vi "IRange Max Min.vi"(1 "resources":i32[](array[numeric])) -> (0 "disabled ranges":i32[](array[numeric]))   [LabVIEW 2022 SP3, in "EClib functions.lvlib"]
doc: "Builds an arrays of indices of the unavailable current ranges."
uses:
  EClib functions.lvlib
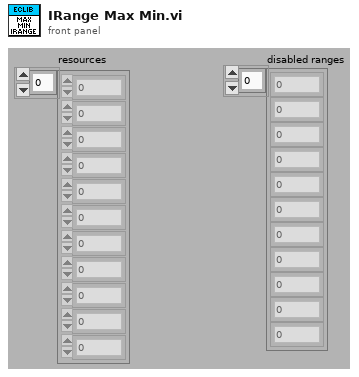
[diagram p1: front panel]
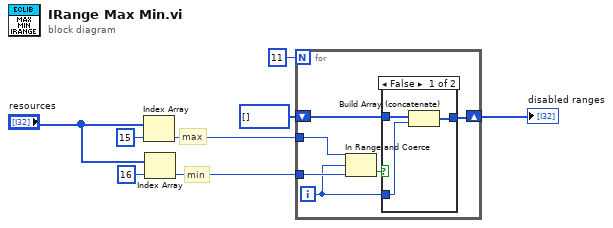
[diagram p0: block diagram]
diagram:
  # "max"
  # "min"
  n1 = Index Array(array="resources", index=15) -> (element=w2:i32)
  n2 = Index Array(array="resources", index=16) -> (element=w1:i32)
  n3 = for {
    N: 11 -> [_]
    tunnel: w2 -> [w14]
    tunnel: w1 -> [w13]
    shift-right: [w11] -> w3
    shift-left: i32[] [] -> [w10]
    i -> [w9]
    n4 = In Range and Coerce(upper limit=w14, x=w9, lower limit=w13) -> (In Range?=w12:bool)  [unwired: 1 out]
    n5 = case shown="False" w12 {
      tunnel: w9 -> [w17 _]
      tunnel: [w16 w18] -> w11
      tunnel: w10 -> [w15 w18]
      frame False {
        n6 = Build Array (concatenate)(w15, w17) -> (w16:i32[])
      }
      frame True {
      }
    }
  }
  "disabled ranges" <- w3
